vi "String.2D Str Array to CSV String.vi"(11 "2D In":string[][](array[string])) -> (3 "spreadsheet string":string)   [LabVIEW 2018]
uses:
  <vilib>/KATE/Files/File Utils.lvlib
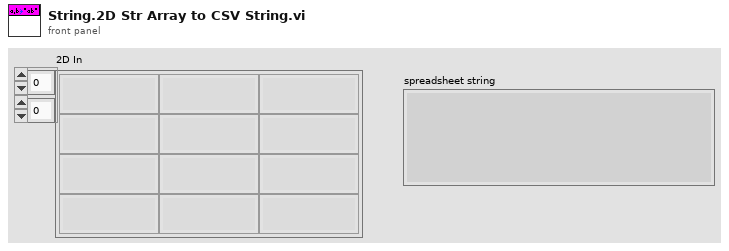
[diagram p1: front panel]
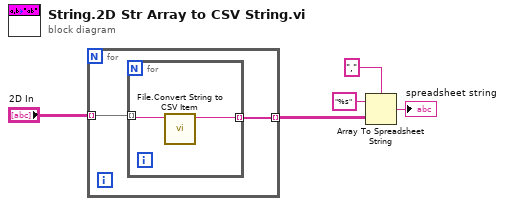
[diagram p0: block diagram]
diagram:
  n1 = for {
    tunnel: "2D In" -> [w7] mode=indexing
    tunnel: [w6] -> w4 mode=indexing
    n2 = for {
      tunnel: w7 -> [w9] mode=indexing
      tunnel: [w8] -> w6 mode=indexing
      n3 = call <vilib>:"File.Convert String to CSV Item.vi"("String"=w9) -> ("String Out"=w8:string)  [unwired: 10 in]
    }
  }
  n4 = Array To Spreadsheet String(delimiter (Tab)=",", array=w4, 3:"%s" ("format string")) -> (spreadsheet string=→"spreadsheet string":string)
